vi "Reorder Variant-Example.vi"() -> ()   [LabVIEW 2015]
uses:
  <vilib>/addons/_JKI.lib/Serialization/JSON/JKI JSON Serialization.lvlib
panel:
  out "data":T1
  in  "Reference Datatype":T2
  out "Output VCluster":variant
  out "error out":errorcluster
  in  "error in (no error)":errorcluster
  in  "JSON String Datatype":string="{\n\"Boolean1\": true,\n\"Double2\": 45.98,\n\"Num1\": 2,\n\"Num2\": 3,\n\"ArrayClusters\": [\n{\n\"name\": \"new\",\n\"num\": 2\n},\n{\n\"num\": 3,\n\"name\": \"old\"\n}\n],\n\"Boolean2\": false,\n\"String2\": 4,\n\"String1\": 5,\n\"Double1\": 3.00\n}"
  # "{\n\"Boolean1\": true,\n\"Double2\": 45.98,\n\"Num1\": 2,\n\"Num2\": 3,\n\"ArrayClusters\": [\n{\n\"name\": \"new\",\n\"num\": 2\n},\n{\n\"num\": 3,\n\"name\": \"old\"\n}\n],\n\"ArrayPrimitive1\": [12,34,54],\n\"ArrayPrimitive2\": [true,false,true,true],\n\"Boolean2\": false,\n\"String2\": 4,\n\"String1\": 5,\n\"Double1\": 3.00,\n\"NegativeNumber\": -67,\n\"Cluster1\": {\n\"num1\": 32,\n\"String1\": \"Tested\",\n\"Cluster12\": {\n\"num12\": 32.43,\n\"String12\": \"Test2\"\n}\n}\n}"
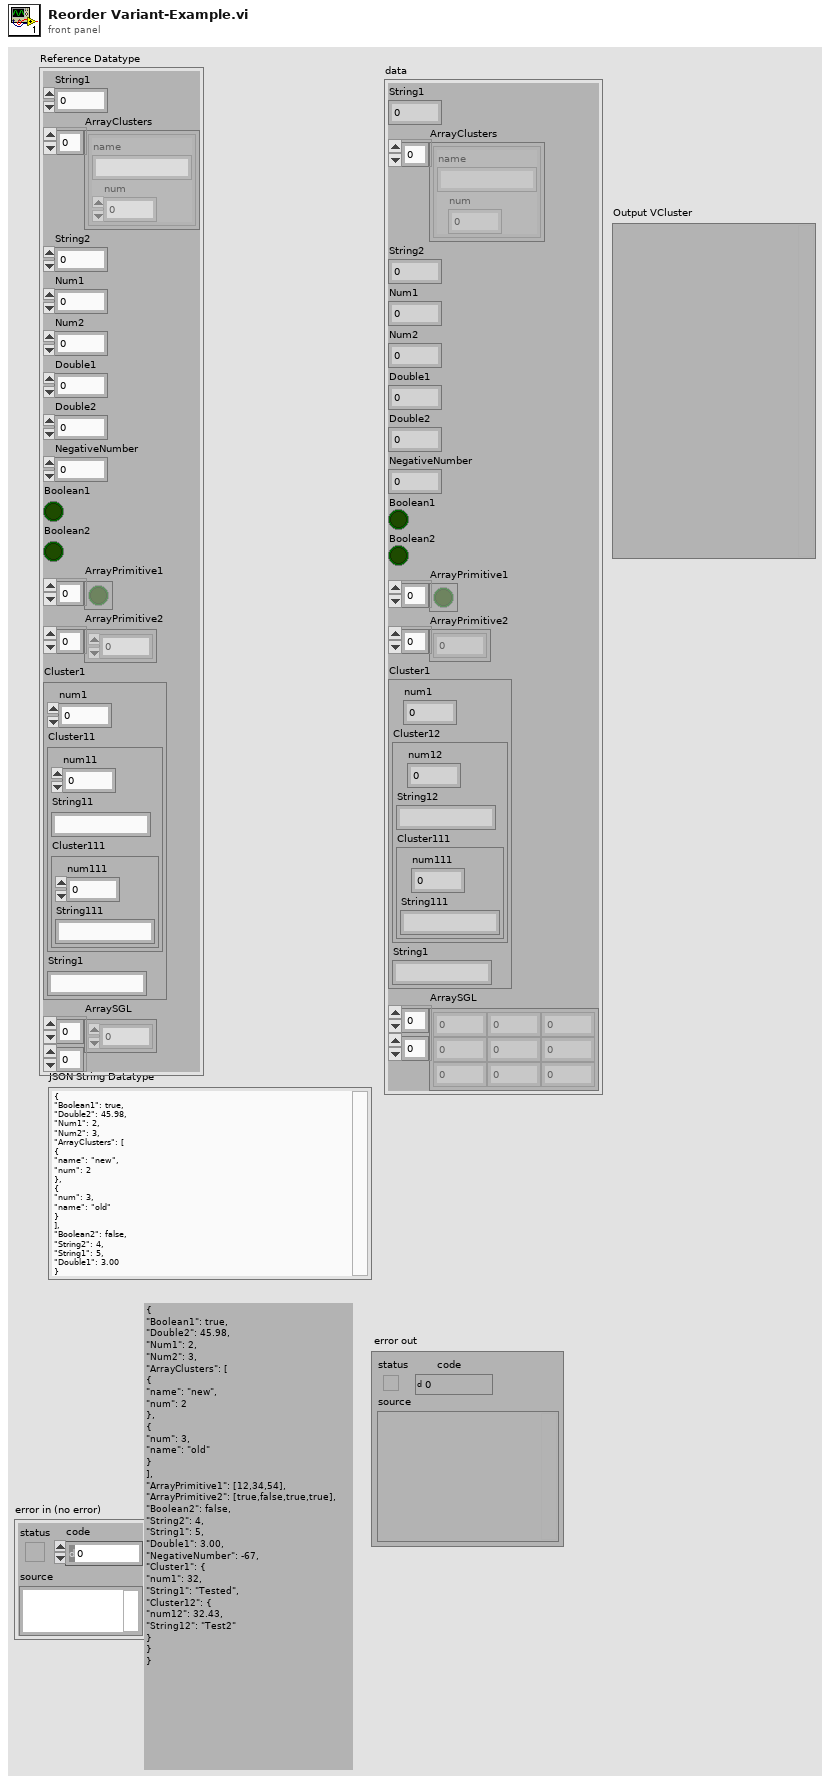
[diagram p1: front panel]
types:
  T1 = cluster{"String1":dbl, "ArrayClusters":cluster{"name":string, "num":dbl}[], "String2":dbl, "Num1":dbl, "Num2":dbl, "Double1":dbl, "Double2":dbl, "NegativeNumber":dbl, "Boolean1":bool, "Boolean2":bool, "ArrayPrimitive1":bool[], "ArrayPrimitive2":dbl[], "Cluster1":cluster{"num1":dbl, "Cluster12":cluster{"num12":dbl, "String12":string, "Cluster111":cluster{"num111":dbl, "String111":string}}, "String1":string}, "ArraySGL":sgl[][]}
  T2 = cluster{"String1":dbl, "ArrayClusters":cluster{"name":string, "num":dbl}[], "String2":dbl, "Num1":dbl, "Num2":dbl, "Double1":dbl, "Double2":dbl, "NegativeNumber":dbl, "Boolean1":bool, "Boolean2":bool, "ArrayPrimitive1":bool[], "ArrayPrimitive2":dbl[], "Cluster1":cluster{"num1":dbl, "Cluster11":cluster{"num11":dbl, "String11":string, "Cluster111":cluster{"num111":dbl, "String111":string}}, "String1":string}, "ArraySGL":sgl[][]}
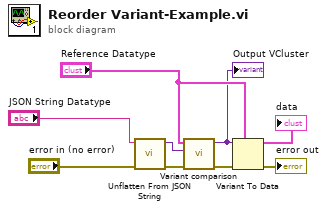
[diagram p0: block diagram]
diagram:
  n1 = call <vilib>:"Unflatten From JSON String.vi"("error in (no error)"="error in (no error)", "JSON String"="JSON String Datatype") -> ("error out"=w7:errorcluster, "Variant"=w6:variant)  [unwired: 8 in]
  n2 = call "Variant comparison.vi"("error in (no error)"=w7, "Data Variant"=w6, "Reference Variant"="Reference Datatype") -> ("error out"=w5:errorcluster, "Output VData"=w2:variant)  [unwired: 7 in]
  "Output VCluster" <- w2
  n3 = Variant To Data(error in=w5, type="Reference Datatype", Variant=w2) -> (data=→"data":T2, error out=→"error out":errorcluster)
